vi "Read remote address.vi"(8 "error in (no error)":errorcluster, 11 "TCP_Streamer in":refnum<class "TCP_Streamer_Publisher.lvclass">) -> (0 "error out":errorcluster, 2 "remote address":string, 3 "TCP_Streamer out":refnum<class "TCP_Streamer_Publisher.lvclass">)   [LabVIEW 2021, in "TCP_Streamer_Publisher.lvclass"]
uses:
  TCP_Streamer_Publisher.lvclass
  TCP_Streamer_Publisher.lvclass/TCP_Streamer_Publisher.ctl
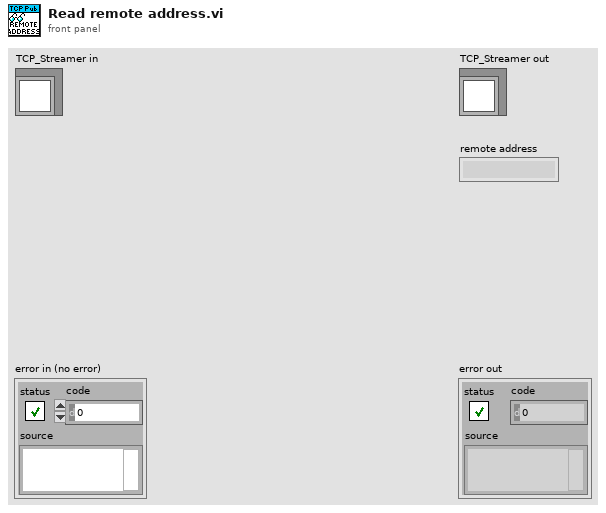
[diagram p1: front panel]
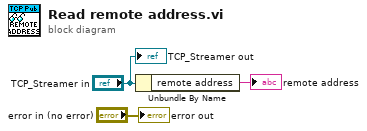
[diagram p0: block diagram]
diagram:
  n1 = Unbundle By Name("TCP_Streamer in") -> ("remote address"=→"remote address":string)
  "error out" <- "error in (no error)"
  "TCP_Streamer out" <- "TCP_Streamer in"
